vi "Unsuppress lines.vi"(8 "error in (no error)":errorcluster, 10 "Lines to unsuppress":u8[](array[numeric]), 11 "TTL in":refnum<class "TTL.lvclass">) -> (0 "error out":errorcluster, 3 "TTL out":refnum<class "TTL.lvclass">)   [LabVIEW 2011, in "TTL.lvclass"]
doc: "This VI restores the original state of lines that were suppressed with the \"Suppress lines\" VI."
uses:
  TTL.lvclass
  TTL.lvclass/TTL.ctl
  <vilib>/DAQmx/write.llb/DAQmx Write (Digital 1D Bool NChan 1Samp 1Line).vi
  <vilib>/DAQmx/read.llb/DAQmx Read (Digital 1D Bool NChan 1Samp 1Line).vi
  <vilib>/DAQmx/miscellaneous.llb/DAQmx Fill In Error Info.vi
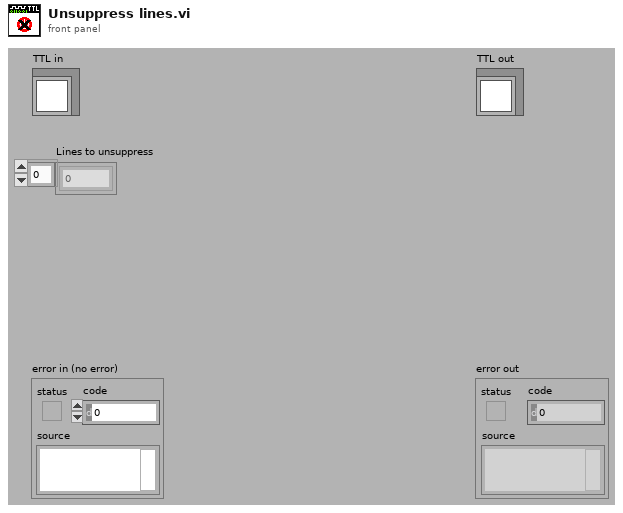
[diagram p1: front panel]
types:
  T1 = typedef "TTL.lvclass/TTL Status Data.ctl" = cluster{"Line states before suppression":bool[], "Suppressed lines":bool[]}
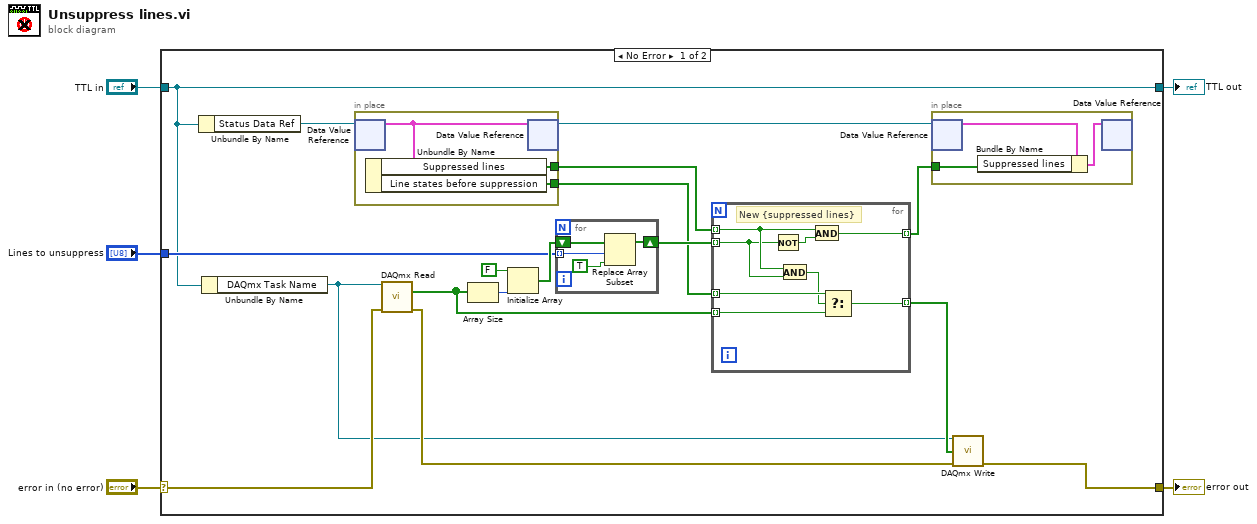
[diagram p0: block diagram]
diagram:
  n1 = case shown="No Error" "error in (no error)" {
    selector: "error in (no error)" -> [w9 w42]
    tunnel: [w22 w42] -> w4
    tunnel: [w15 w41] -> w2
    tunnel: "TTL in" -> [w15 w41]
    tunnel: "Lines to unsuppress" -> [w17 _]
    frame No Error {
      n2 = Unbundle By Name(w15) -> ("Status Data Ref"=w14:refnum<data-value>)
      n3 = Unbundle By Name(w15) -> ("DAQmx Task Name"=w6:refnum<k21>)
      n4 = in-place {
        in-place-border: [w27] -> w13
        in-place-border: [w26] -> w12
        n5 = in-place-dvr #1(w14) -> (w28:T1)  [unwired: 1 out]
        n6 = Unbundle By Name(w28) -> ("Suppressed lines"=w27:bool[], "Line states before suppression"=w26:bool[])
        n7 = in-place-dvr #1(w28) -> (w10:refnum<data-value>)  [unwired: 1 out]
      }
      n8 = call-poly <vilib>:"DAQmx Read.vi"("task/channels in"=w6, "error in"=w9) -> ("data"=w7:bool[], "error out"=w8:errorcluster)  [unwired: 11 in, 1 out]
      n9 = Array Size(array=w7) -> (size(s)=w20:i32)
      n10 = Initialize Array(FALSE, w20) -> (w18:bool[])
      n11 = for {
        shift-right: [w31] -> w16
        shift-left: w18 -> [w32]
        tunnel: w17 -> [w30] mode=indexing
        n12 = Replace Array Subset(array=w32, new element=TRUE, index=w30) -> (w31:bool[])
      }
      n13 = for {
        tunnel: w13 -> [w36] mode=indexing
        tunnel: w7 -> [w38] mode=indexing
        tunnel: w12 -> [w37] mode=indexing
        tunnel: w16 -> [w35] mode=indexing
        tunnel: [w39] -> w11 mode=indexing
        tunnel: [w33] -> w21 mode=indexing
        # "New {suppressed lines}"
        n14 = Not(x=w35) -> (.not. x?=w40:bool)
        n15 = And(x=w36, y=w35) -> (x .and. y?=w34:bool)
        n16 = And(x=w36, y=w40) -> (x .and. y?=w39:bool)
        n17 = Select(t=w37, s=w34, f=w38) -> (s? t:f=w33:bool)
      }
      n18 = in-place {
        in-place-border: w11 -> [w23]
        n19 = in-place-dvr #2(w10) -> (w25:T1)  [unwired: 1 out]
        n20 = Bundle By Name(cluster=w25, "Suppressed lines"=w23) -> (w24:T1)
        n21 = in-place-dvr #2(w24) -> ()  [unwired: 2 out]
      }
      n22 = call-poly <vilib>:"DAQmx Write.vi"("task/channels in"=w6, "data"=w21, "error in"=w8) -> ("error out"=w22:errorcluster)  [unwired: 10 in, 2 out]
    }
    frame Error {
    }
  }
  "error out" <- w4
  "TTL out" <- w2
